vi "I32ToI16.vi"(5 "Number":i32) -> (1 "Signed 16-bit integer":i16, 2 "Overflow?":bool, 3 "Exact conversion?":bool)   [LabVIEW 2017, in "GPOverflow.lvlib"]
doc: "Converts <B>Number</B> to I16 keeping track of numeric overflow and exactness of conversion.\n\n<B>Exact conversion?</B> will be True only if a conversion back into the original data type of <B>Number</B> will yield the exact same number, i.e. no precision was lost during the conversion.\n\n<B>Overflow?</B> will be True if positive or negative overflow occurred. The numeric output will saturate in case of overflow.\n\nThis VI is inlined.\n\nSteen Schmidt\nGPower\n6/3 2013"
uses:
  GPOverflow.lvlib
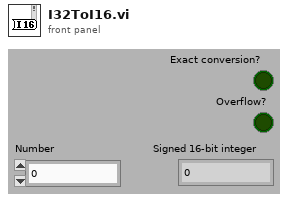
[diagram p1: front panel]
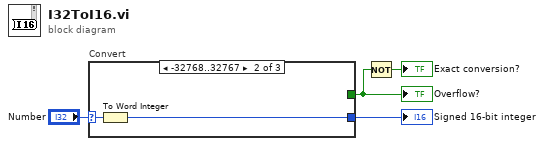
[diagram p0: block diagram]
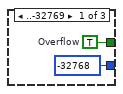
[diagram p2: hidden frame]
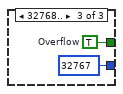
[diagram p3: hidden frame]
diagram:
  n1 = case "Convert" shown="-32768..32767" "Number" {
    selector: "Number" -> [_ w8 _]
    tunnel: [i16 -32768 w7 i16 32767] -> w3
    tunnel: [w5 _ w9] -> w2
    frame ..-32769 {
      w5 = TRUE  # Overflow
    }
    frame -32768..32767 {
      n2 = To Word Integer(number=w8) -> (16bit integer=w7:i16)
    }
    frame 32768.. {
      w9 = TRUE  # Overflow
    }
  }
  "Signed 16-bit integer" <- w3
  "Overflow?" <- w2
  n3 = Not(x=w2) -> (.not. x?=→"Exact conversion?":bool)
